vi "Initial.vi"(8 "error in (no error)":errorcluster, 11 "ZanClass in":refnum<class "ZanClass.lvclass">) -> (0 "error out":errorcluster, 3 "ZanClass out":refnum<class "ZanClass.lvclass">)   [LabVIEW 2019, in "ZanClass.lvclass"]
uses:
  ZanClass.lvclass
  LLB/zmotion/zaux/zauxdll.lvlib
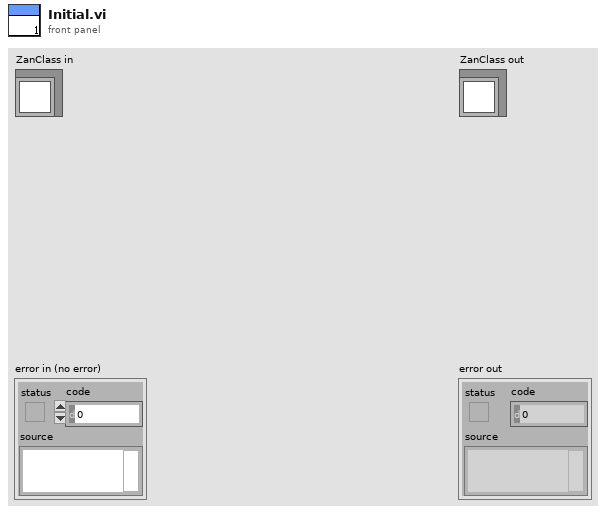
[diagram p1: front panel]
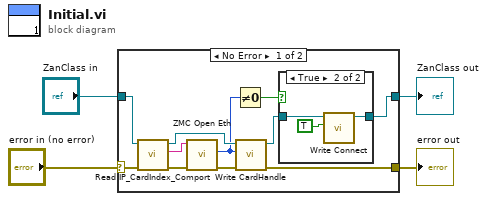
[diagram p0: block diagram]
diagram:
  n1 = case shown="No Error" "error in (no error)" {
    selector: "error in (no error)" -> [w13 w20]
    tunnel: "ZanClass in" -> [w15 w21]
    tunnel: [w9 w21] -> w2
    tunnel: [w8 w20] -> w1
    frame No Error {
      n2 = call-dynamic "Read IP_CardIndex_Comport.vi"("error in (no error)"=w13, "AxisCard in"=w15) -> ("error out"=w12:errorcluster, "IP/CardIndex/Comport"=w5:string, "AxisCard out"=w14:refnum<class "ZanClass.lvclass">)  [unwired: 7 in]
      n3 = call "ZMC Open Eth.vi"("error in (no error)"=w12, "ipaddr"=w5) -> ("error out"=w11:errorcluster, "phandle out"=w6:u32)  [unwired: 6 in, 2 out]
      n4 = Not Equal To 0?(x=w6) -> (x != 0?=w7:bool)
      n5 = call-dynamic "Write CardHandle.vi"("error in (no error)"=w11, "CardHandle"=w6, "AxisCard in"=w14) -> ("error out"=w8:errorcluster, "AxisCard out"=w10:refnum<class "ZanClass.lvclass">)  [unwired: 7 in]
      n6 = case shown="True" w7 {
        tunnel: w10 -> [w16 w19]
        tunnel: [w16 w18] -> w9
        frame False {
        }
        frame True {
          n7 = call-dynamic "Write Connect.vi"("Connect"=TRUE, "AxisCard in"=w19) -> ("AxisCard out"=w18:refnum<class "ZanClass.lvclass">)  [unwired: 8 in, 1 out]
        }
      }
    }
    frame Error {
    }
  }
  "error out" <- w1
  "ZanClass out" <- w2
